vi "AlliGator Variable Names.vi"() -> (0 "Sorted Index Array":i32[](array[numeric]), 1 "Sorted Variable Internal Names":string[](array[string]), 2 "Sorted Basic Variable Names":string[](array[string]), 3 "Basic Variable Names":string[](array[string]))   [LabVIEW 2021, in "AlliGator Phasor Plot.lvlib"]
doc: "Stores basic variable names and their internal counterparts (used in formula)."
uses:
  AlliGator Phasor Plot.lvlib
  <userlib>/_OpenG.lib/array/array.llb/Sort 1D Array (I32)__ogtk.vi
  <userlib>/_OpenG.lib/array/array.llb/Reorder 1D Array2 (String)__ogtk.vi
  <userlib>/_OpenG.lib/array/array.llb/openg_array.lvlib
panel:
  # "see the AlliGator License on the block diagram (Ctrl+E or Window:Show Block Diagram)"
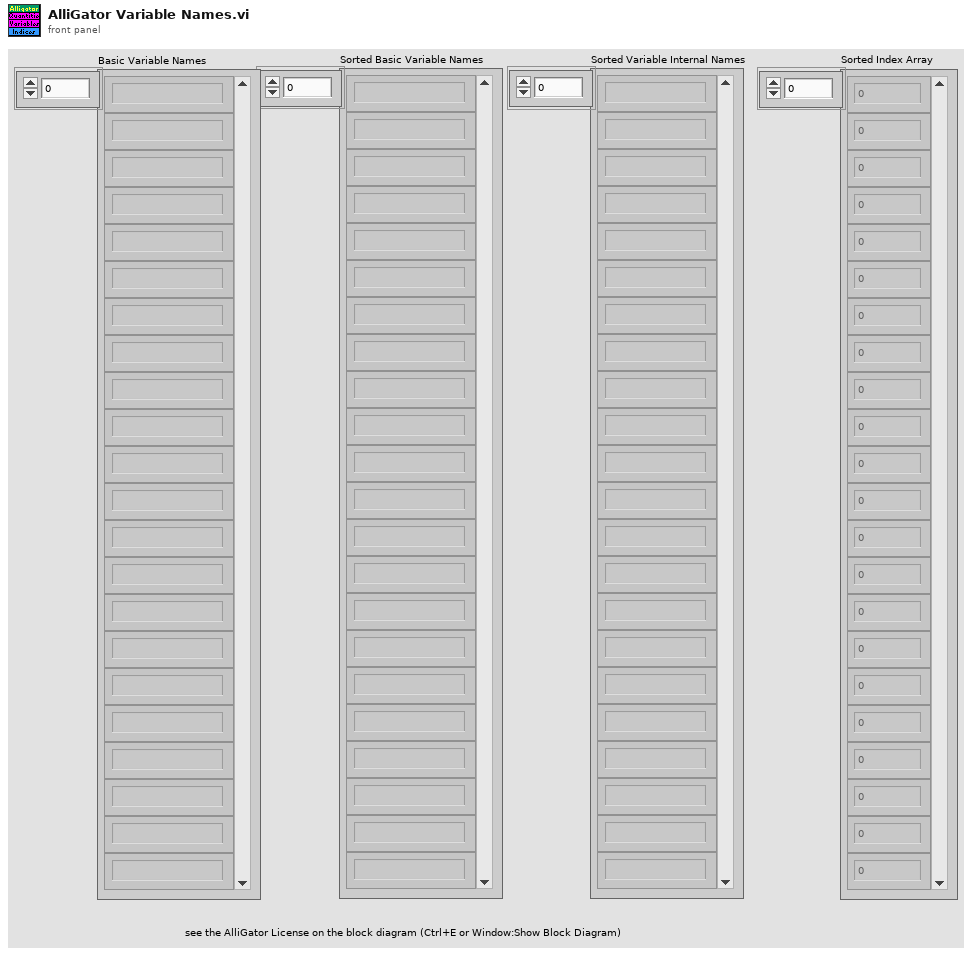
[diagram p1: front panel]
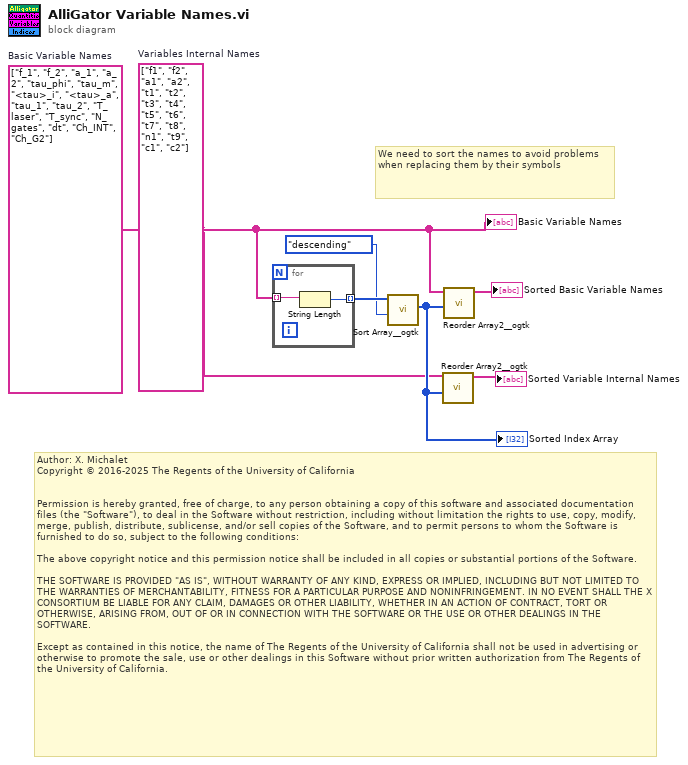
[diagram p0: block diagram]
diagram:
  w1 = string[] ["f1", "f2", "a1", "a2", "t1", "t2", "t3", "t4", "t5", "t6", "t7", "t8", "n1", "t9", "c1", "c2"]  # Variables Internal Names
  w2 = string[] ["f_1", "f_2", "a_1", "a_2", "tau_phi", "tau_m", "<tau>_i", "<tau>_a", "tau_1", "tau_2", "T_laser", "T_sync", "N_gates", "dt", "Ch_INT", "Ch_G2"]  # Basic Variable Names
  # "Author: X. Michalet\nCopyright © 2016-2025 The Regents of the University of California\n \n\nPermission is hereby granted, free of charge, to any person obtaining a copy of this software and associated documentation files (the \"Software\"), to deal in the Software without restriction, including without limitation the rights to use, copy, modify, merge, publish, distribute, sublicense, and/or sell copies of the Software, and to permit persons to whom the Software is furnished to do so, subject to the following conditions:\n\nThe above copyright notice and this permission notice shall be included in all copies or substantial portions of the Software.\n\nTHE SOFTWARE IS PROVIDED \"AS IS\", WITHOUT WARRANTY OF ANY KIND, EXPRESS OR IMPLIED, INCLUDING BUT NOT LIMITED TO THE WARRANTIES OF MERCHANTABILITY, FITNESS FOR A PARTICULAR PURPOSE AND NONINFRINGEMENT. IN NO EVENT SHALL THE X CONSORTIUM BE LIABLE FOR ANY CLAIM, DAMAGES OR OTHER LIABILITY, WHETHER IN AN ACTION OF CONTRACT, TORT OR OTHERWISE, ARISING FROM, OUT OF OR IN CONNECTION WITH THE SOFTWARE OR THE USE OR OTHER DEALINGS IN THE SOFTWARE.\n\nExcept as contained in this notice, the name of The Regents of the University of California shall not be used in advertising or otherwise to promote the sale, use or other dealings in this Software without prior written authorization from The Regents of the University of California."
  # "We need to sort the names to avoid problems when replacing them by their symbols"
  n1 = for {
    tunnel: w2 -> [w9] mode=indexing
    tunnel: [w8] -> w7 mode=indexing
    n2 = String Length(string=w9) -> (length=w8:i32)
  }
  n3 = call-poly <userlib>:"Sort Array__ogtk.vi"("Order"=enum16{"ascending", "descending"}."descending", "Array in"=w7) -> ("Sorted Pointers"=w3:i32[])  [unwired: 8 in, 1 out]
  "Sorted Index Array" <- w3
  n4 = call-poly <userlib>:"Reorder Array2__ogtk.vi"("indices"=w3, "array"=w1) -> ("reordered array"=→"Sorted Variable Internal Names":string[])  [unwired: 9 in]
  n5 = call-poly <userlib>:"Reorder Array2__ogtk.vi"("indices"=w3, "array"=w2) -> ("reordered array"=→"Sorted Basic Variable Names":string[])  [unwired: 9 in]
  "Basic Variable Names" <- w2
